vi "bulk_read_write.vi"() -> ()   [LabVIEW 2015]
uses:
  dxl_x86_c.lvlib/dxl_x86_c.lvlib
panel:
  in  "value : PRO (slide)\nLED RED":bool
  in  "LEN_PRO_\nGOAL_POSITION":u16=4
  out "groupwrite_num":i32
  in  "LEN_PRO_\nLED_RED":u16=1
  in  "ADDR_PRO_\nLED_RED":u16=563
  out "value : PRO (LED)\nLED_RED":bool
  out "groupread_num":i32
  in  "LEN_PRO_\nPRESENT_POSITION":u16=4
  in  "dynamixe2_id":u8=2
  in  "device_name":string="COM1"
  in  "ADDR_PRO_\nPRESENT_POSITION":u16=611
  in  "ADDR_PRO_\nGOAL_POSITION":u16=596
  in  "ADDR_PRO_\nTORQUE_ENABLE":u16=562
  out "protocol_version":dbl=2.0
  out "value : PRO (knob)\npresent position 1":i32(knob) scale=150000.0..-150000.0
  in  "terminate":bool
  out "port_num":i32
  in  "value : PRO (dial)\ngoal position":i32(knob) scale=150000.0..-150000.0
  in  "dynamixel1_id":u8=1
  in  "baud_rate":i32=1000000
  # "bulk_read_write.vi\n\nCreated on: 2016. 6. 13\nAuthor: Ryu Woon Jung (Leon)\n\n*********     Bulk Read and Bulk Write Example      *********\n\n\nAvailable DXL model on this example : All models using Protocol 2.0\nThis example is designed for using two Dynamixel PRO 54-200, and an USB2DYNAMIXEL.\nTo use another Dynamixel model, such as X series, see their details in E-Manual(support.robotis.com) \n   and edit \"numeric control\"s seen left with \"Edit Text\" tool.\nBe sure that Dynamixel PRO properties are already set as %% ID : 1 / Baudnum : 3 (Baudrate : 1000000 [1M])\n\n1. Run example by click above \"Run\" button (below \"Edit\" menu).\n2. Drag \"dial\" then you may see the Dynamixel and \"knob\"s rotating\n3. Click \"slide button\" then you may see the LED of Dynamixel lighting\n4. To finish the example, press \"terminate\" button."
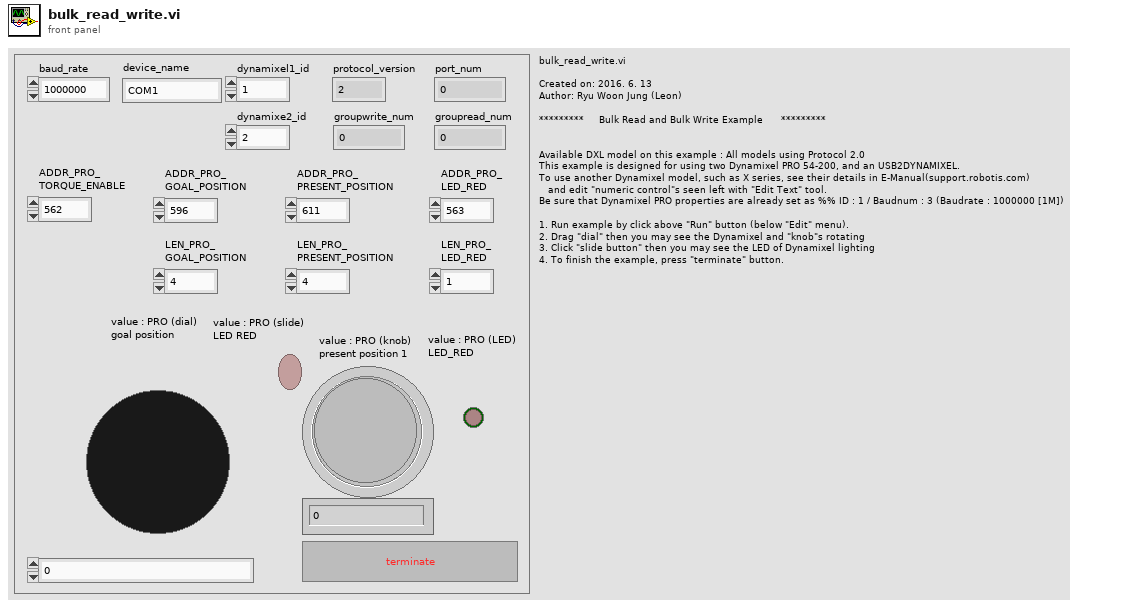
[diagram p1: front panel]
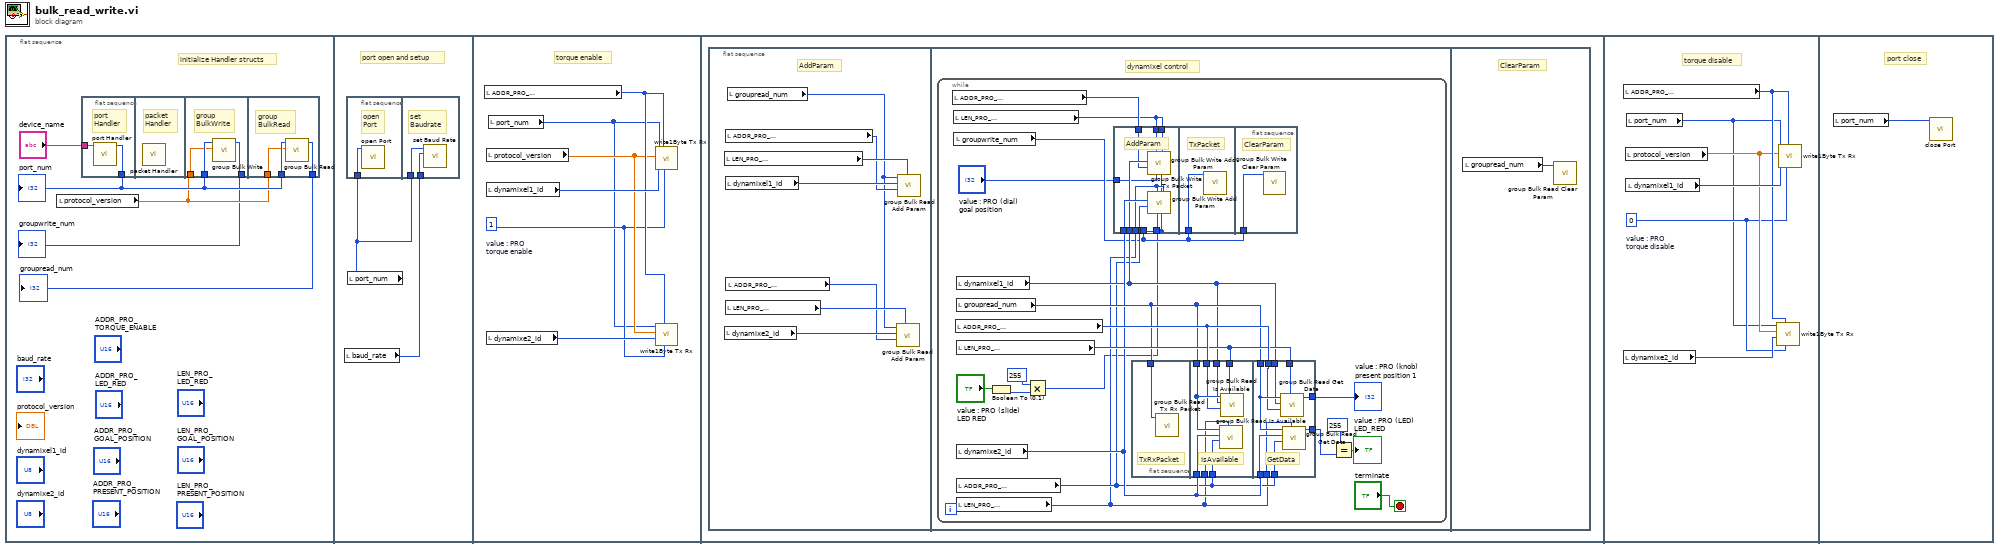
[diagram p0: block diagram]
diagram:
  n1 = flat-sequence {
    frame #0 {
      # "initialize Handler structs"
      n2 = local read "protocol_version"() -> (w3:dbl)
      n3 = flat-sequence {
        tunnel: "device_name" -> [w7]
        tunnel: [w6] -> w4
        tunnel: w3 -> [w8]
        tunnel: w4 -> [w10]
        tunnel: [w9] -> w2
        tunnel: w4 -> [w13]
        tunnel: w3 -> [w12]
        tunnel: [w11] -> w1
        frame #0 {
          # "port\nHandler"
          n4 = call "port Handler.vi"("port_name"=w7) -> ("function return"=w6:i32)  [unwired: 10 in]
        }
        frame #1 {
          # "packet\nHandler"
          n5 = call "packet Handler.vi"() -> ()  [unwired: 12 in]
        }
        frame #2 {
          # "group\nBulkWrite"
          n6 = call "group Bulk Write.vi"("protocol_version"=w8, "port_num"=w10) -> ("function return"=w9:i32)  [unwired: 9 in]
        }
        frame #3 {
          # "group\nBulkRead"
          n7 = call "group Bulk Read.vi"("protocol_version"=w12, "port_num"=w13) -> ("function return"=w11:i32)  [unwired: 9 in]
        }
      }
      "port_num" <- w4
      "groupread_num" <- w1
      "groupwrite_num" <- w2
    }
    frame #1 {
      # "port open and setup"
      n8 = local read "baud_rate"() -> (w14:i32)
      n9 = flat-sequence {
        tunnel: w15 -> [w16]
        tunnel: w15 -> [w18]
        tunnel: w14 -> [w17]
        frame #0 {
          # "open\nPort"
          n10 = call "open Port.vi"("port_num"=w16) -> ()  [unwired: 10 in, 1 out]
        }
        frame #1 {
          # "set\nBaudrate"
          n11 = call "set Baud Rate.vi"("baudrate"=w17, "port_num"=w18) -> ()  [unwired: 9 in, 1 out]
        }
      }
      n12 = local read "port_num"() -> (w15:i32)
    }
    frame #2 {
      w20 = 1  # value : PRO torque enable
      # "torque enable"
      n13 = local read "ADDR_PRO_\nTORQUE_ENABLE"() -> (w23:u16)
      n14 = local read "protocol_version"() -> (w22:dbl)
      n15 = local read "dynamixel1_id"() -> (w24:u8)
      n16 = local read "dynamixe2_id"() -> (w21:u8)
      n17 = local read "port_num"() -> (w19:i32)
      n18 = call "write1Byte Tx Rx.vi"("data"=w20, "address"=w23, "id"=w24, "protocol_version"=w22, "port_num"=w19) -> ()  [unwired: 7 in]
      n19 = call "write1Byte Tx Rx.vi"("data"=w20, "address"=w23, "id"=w21, "protocol_version"=w22, "port_num"=w19) -> ()  [unwired: 7 in]
    }
    frame #3 {
      n20 = flat-sequence {
        frame #0 {
          # "AddParam"
          n21 = local read "LEN_PRO_\nPRESENT_POSITION"() -> (w31:u16)
          n22 = local read "dynamixe2_id"() -> (w26:u8)
          n23 = local read "ADDR_PRO_\nPRESENT_POSITION"() -> (w29:u16)
          n24 = local read "dynamixel1_id"() -> (w30:u8)
          n25 = local read "LEN_PRO_\nLED_RED"() -> (w28:u16)
          n26 = local read "ADDR_PRO_\nLED_RED"() -> (w25:u16)
          n27 = local read "groupread_num"() -> (w27:i32)
          n28 = call "group Bulk Read Add Param.vi"("data_length"=w28, "start_address"=w25, "id"=w26, "group_num"=w27) -> ()  [unwired: 7 in, 1 out]
          n29 = call "group Bulk Read Add Param.vi"("data_length"=w31, "start_address"=w29, "id"=w30, "group_num"=w27) -> ()  [unwired: 7 in, 1 out]
        }
        frame #1 {
          # "dynamixel control"
          n30 = while {
            stop <- "terminate" stop-if-true
            n31 = local read "ADDR_PRO_\nGOAL_POSITION"() -> (w40:u16)
            n32 = local read "LEN_PRO_\nGOAL_POSITION"() -> (w39:u16)
            n33 = local read "groupwrite_num"() -> (w37:i32)
            n34 = local read "ADDR_PRO_\nPRESENT_POSITION"() -> (w50:u16)
            n35 = local read "dynamixel1_id"() -> (w43:u8)
            n36 = local read "groupread_num"() -> (w45:i32)
            n37 = local read "LEN_PRO_\nPRESENT_POSITION"() -> (w46:u16)
            n38 = local read "dynamixe2_id"() -> (w44:u8)
            n39 = local read "ADDR_PRO_\nLED_RED"() -> (w42:u16)
            n40 = local read "LEN_PRO_\nLED_RED"() -> (w41:u16)
            n41 = Boolean To (0,1)(Boolean="value : PRO (slide)\nLED RED") -> (0, 1=w34:i16)
            n42 = Multiply(x=255, y=w34) -> (x*y=w33:i32)
            n43 = flat-sequence {
              tunnel: [w52] -> _
              tunnel: w44 -> [w61]
              tunnel: w43 -> [w60]
              tunnel: w42 -> [w59]
              tunnel: w41 -> [w55]
              tunnel: w40 -> [w58]
              tunnel: w39 -> [w57]
              tunnel: w39 -> [w56]
              tunnel: "value : PRO (dial)\ngoal position" -> [w54]
              tunnel: w33 -> [w53]
              tunnel: w37 -> [w52]
              tunnel: w37 -> [w62]
              tunnel: w37 -> [w63]
              frame #0 {
                # "AddParam"
                n44 = call "group Bulk Write Add Param.vi"("input_length"=w56, "data"=w54, "data_length"=w57, "start_address"=w58, "id"=w60, "group_num"=w52) -> ()  [unwired: 5 in, 1 out]
                n45 = call "group Bulk Write Add Param.vi"("input_length"=w55, "data"=w53, "data_length"=w55, "start_address"=w59, "id"=w61, "group_num"=w52) -> ()  [unwired: 5 in, 1 out]
              }
              frame #1 {
                # "TxPacket"
                n46 = call "group Bulk Write Tx Packet.vi"("group_num"=w62) -> ()  [unwired: 11 in]
              }
              frame #2 {
                # "ClearParam"
                n47 = call "group Bulk Write Clear Param.vi"("group_num"=w63) -> ()  [unwired: 11 in]
              }
            }
            n48 = flat-sequence {
              tunnel: w45 -> [w64]
              tunnel: w45 -> [w71]
              tunnel: w44 -> [w70]
              tunnel: w50 -> [w69]
              tunnel: w41 -> [w68]
              tunnel: w42 -> [w67]
              tunnel: w46 -> [w66]
              tunnel: w43 -> [w65]
              tunnel: w45 -> [w80]
              tunnel: w44 -> [w79]
              tunnel: w50 -> [w78]
              tunnel: w41 -> [w75]
              tunnel: [w77] -> w35
              tunnel: [w76] -> w47
              tunnel: w42 -> [w74]
              tunnel: w46 -> [w73]
              tunnel: w43 -> [w72]
              frame #0 {
                # "TxRxPacket"
                n49 = call "group Bulk Read Tx Rx Packet.vi"("group_num"=w64) -> ()  [unwired: 11 in]
              }
              frame #1 {
                # "IsAvailable"
                n50 = call "group Bulk Read Is Available.vi"("data_length"=w68, "address"=w67, "id"=w70, "group_num"=w71) -> ()  [unwired: 7 in, 1 out]
                n51 = call "group Bulk Read Is Available.vi"("data_length"=w66, "address"=w69, "id"=w65, "group_num"=w71) -> ()  [unwired: 7 in, 1 out]
              }
              frame #2 {
                # "GetData"
                n52 = call "group Bulk Read Get Data.vi"("data_length"=w73, "address"=w78, "id"=w72, "group_num"=w80) -> ("function return"=w76:u32)  [unwired: 7 in]
                n53 = call "group Bulk Read Get Data.vi"("data_length"=w75, "address"=w74, "id"=w79, "group_num"=w80) -> ("function return"=w77:u32)  [unwired: 7 in]
              }
            }
            n54 = Equal?(x=255, y=w35) -> (x = y?=→"value : PRO (LED)\nLED_RED":bool)
            "value : PRO (knob)\npresent position 1" <- w47
          }
        }
        frame #2 {
          # "ClearParam"
          n55 = local read "groupread_num"() -> (w81:i32)
          n56 = call "group Bulk Read Clear Param.vi"("group_num"=w81) -> ()  [unwired: 11 in]
        }
      }
    }
    frame #4 {
      w83 = 0  # value : PRO torque disable
      # "torque disable"
      n57 = local read "ADDR_PRO_\nTORQUE_ENABLE"() -> (w86:u16)
      n58 = local read "dynamixe2_id"() -> (w84:u8)
      n59 = local read "protocol_version"() -> (w85:dbl)
      n60 = local read "dynamixel1_id"() -> (w87:u8)
      n61 = local read "port_num"() -> (w82:i32)
      n62 = call "write1Byte Tx Rx.vi"("data"=w83, "address"=w86, "id"=w84, "protocol_version"=w85, "port_num"=w82) -> ()  [unwired: 7 in]
      n63 = call "write1Byte Tx Rx.vi"("data"=w83, "address"=w86, "id"=w87, "protocol_version"=w85, "port_num"=w82) -> ()  [unwired: 7 in]
    }
    frame #5 {
      # "port close"
      n64 = local read "port_num"() -> (w88:i32)
      n65 = call "close Port.vi"("port_num"=w88) -> ()  [unwired: 11 in]
    }
  }
